vi "Set Resource.vi"(8 "error in (no error)":errorcluster, 9 "resource info":variant, 10 "name in bitfile":string, 11 "Datatype group in":refnum<class "Datatype group.lvclass">) -> (0 "error out":errorcluster, 2 "replaced":bool, 3 "Datatype group out":refnum<class "Datatype group.lvclass">)   [LabVIEW 2016, in "FPGA RM Shared API.lvlib" / "Datatype group.lvclass"]
uses:
  Datatype group.lvclass
  Datatype group.lvclass/Datatype group.ctl
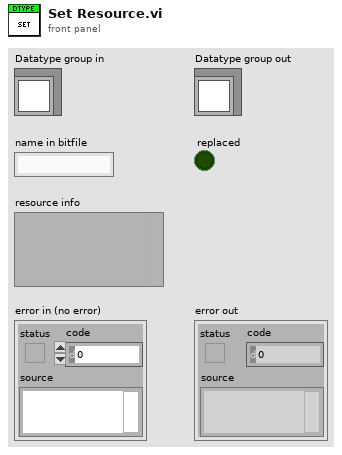
[diagram p1: front panel]
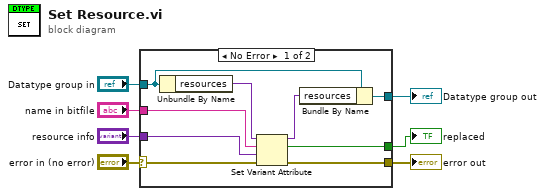
[diagram p0: block diagram]
diagram:
  n1 = case shown="No Error" "error in (no error)" {
    selector: "error in (no error)" -> [w12 w18]
    tunnel: [w11 w18] -> w6
    tunnel: [w13 w17] -> w4
    tunnel: "Datatype group in" -> [w15 w17]
    tunnel: "name in bitfile" -> [w10 _]
    tunnel: "resource info" -> [w9 _]
    tunnel: [w8 _] -> w1
    frame No Error {
      n2 = Unbundle By Name(w15) -> ("resources"=w16:variant)
      n3 = Set Variant Attribute(Variant=w16, name=w10, value=w9, error in=w12) -> (Variant out=w14:variant, replaced=w8:bool, error out=w11:errorcluster)
      n4 = Bundle By Name(cluster=w15, "resources"=w14) -> (w13:refnum<class "Datatype group.lvclass">)
    }
    frame Error {
    }
  }
  "error out" <- w6
  "Datatype group out" <- w4
  "replaced" <- w1
